vi "new cell.vi"(9 "Justification":enum16{"Left", "Center", "Right"}(ring), 10 "BG color":u32(colorbox)=16777216, 11 "String":string) -> (3 "cell":T1)   [LabVIEW 2021, in "RocketPlot.lvlib" / "TipTablePanel.lvclass"]
uses:
  TipTablePanel.lvclass
  cell cache.ctl
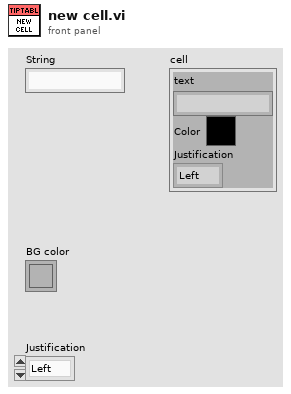
[diagram p1: front panel]
types:
  T1 = typedef "RocketPlot.lvlib/TipTablePanel.lvclass/cell cache.ctl" = cluster{"text":string, "Color":u32, "Justification":enum16{"Left", "Center", "Right"}}
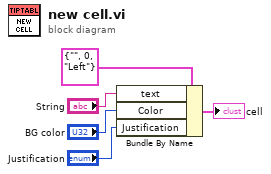
[diagram p0: block diagram]
diagram:
  n1 = Bundle By Name(cluster=T1 {"text"="", "Color"=0, "Justification"=enum."Left"} ("Cluster"), "text"="String", "Color"="BG color", "Justification"="Justification") -> (→"cell":T1)
